vi "Prompt.vi"(8 "error in (no error)":errorcluster, 9 "Default Value":string, 10 "Prompt":string) -> (0 "error out":errorcluster, 1 "Value":string)   [LabVIEW 2017, in "MGI-Console.lvlib" / "Console.lvclass"]
doc: "Prompts the user for input.\n\n<b>Default Value</b> is returned if the user does not enter any input (meaning they just press the enter key).\n----\nCopyright: MGI 2018\nAuthor: Derek Trepanier"
uses:
  Console.lvclass
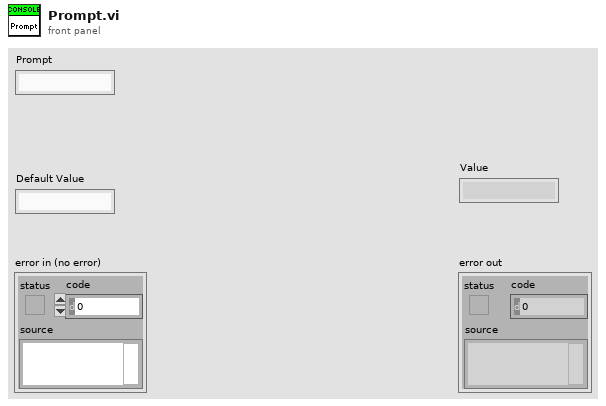
[diagram p1: front panel]
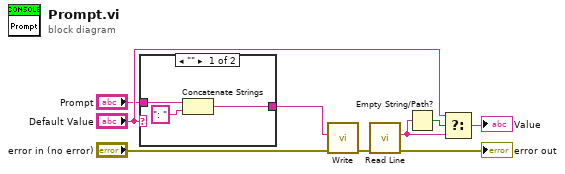
[diagram p0: block diagram]
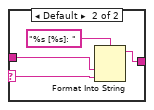
[diagram p2: hidden frame]
diagram:
  n1 = case shown="\"\"" "Default Value" {
    selector: "Default Value" -> [_ w14]
    tunnel: [w11 w15] -> w9
    tunnel: "Prompt" -> [w12 w13]
    frame "" {
      n2 = Concatenate Strings(w12, ": " ("string")) -> (w11:string)
    }
    frame Default {
      n3 = Format Into String(format string="%s [%s]: ", w13, w14) -> (resulting string=w15:string)  [unwired: 2 in, 1 out]
    }
  }
  n4 = call "Write.vi"("error in (no error)"="error in (no error)", "String"=w9) -> ("error out"=w7:errorcluster)  [unwired: 9 in]
  n5 = call "Read Line.vi"("error in (no error)"=w7) -> ("error out"=→"error out":errorcluster, "ReadLine"=w4:string)  [unwired: 9 in]
  n6 = Empty String/Path?(string/path=w4) -> (empty?=w6:bool)
  n7 = Select(t="Default Value", s=w6, f=w4) -> (s? t:f=→"Value":string)
